vi "read_timing_array.vi"(4 "error in":errorcluster, 7 "VISA resource in":refnum<visa-resource-name>) -> (0 "error out 2":errorcluster, 1 "delay array":dbl[](array[numeric]), 3 "VISA resource out":refnum<visa-resource-name>)   [LabVIEW 2011]
doc: "Reads all delay values stored in the DG645 and returns them in an array, from t0 to H.\nSee DG645 documentation for mor info."
panel:
  in  "bytes to read":u32=256
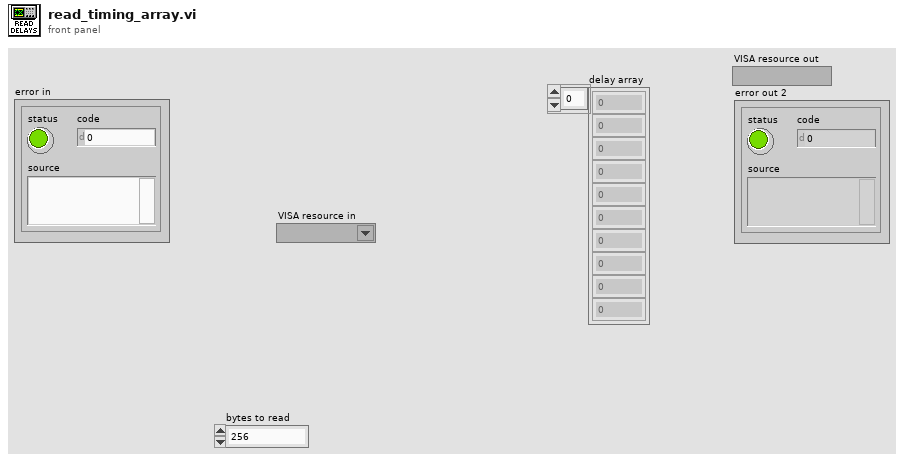
[diagram p1: front panel]
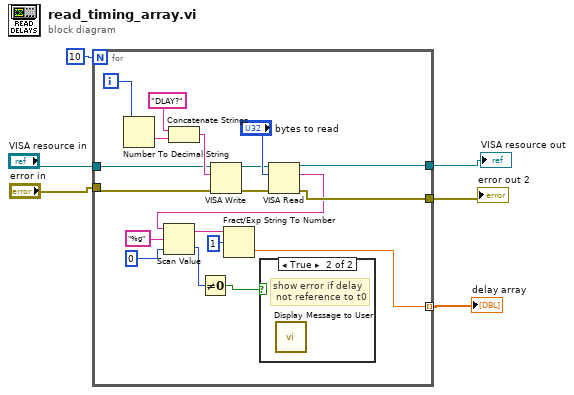
[diagram p0: block diagram]
diagram:
  n1 = for {
    N: 10 -> [_]
    tunnel: "error in" -> [w22]
    tunnel: [w19] -> w5 mode=indexing
    tunnel: [w16] -> w1
    tunnel: "VISA resource in" -> [w11]
    tunnel: [w10] -> w2
    i -> [w9]
    n2 = Number To Decimal String(number=w9) -> (decimal integer string=w18:string)  [unwired: 1 in]
    n3 = Concatenate Strings("DLAY?" ("string"), w18) -> (w17:string)
    n4 = VISA Write(VISA resource name=w11, write buffer=w17, error in (no error)=w22) -> (VISA resource name out=w24:refnum<visa-resource-name>, error out=w23:errorcluster)  [unwired: 1 out]
    n5 = VISA Read(VISA resource name=w24, byte count="bytes to read", error in (no error)=w23) -> (VISA resource name out=w10:refnum<visa-resource-name>, read buffer=w8:string, error out=w16:errorcluster)  [unwired: 1 out]
    n6 = Scan Value(string=w8, format string="%g", default (0 dbl)=u16 0) -> (output string=w13:string, value=w12:u16)
    n7 = Not Equal To 0?(x=w12) -> (x != 0?=w7:bool)
    n8 = Fract/Exp String To Number(string=w13, offset=1) -> (number=w19:dbl)  [unwired: 2 in, 1 out]
    n9 = case shown="True" w7 {
      frame False {
      }
      frame True {
        # "show error if delay\n not reference to t0"
        n10 = call "Display Message to User"() -> ()  [unwired: 10 in, 2 out]
      }
    }
  }
  "delay array" <- w5
  "VISA resource out" <- w2
  "error out 2" <- w1
